vi "Build IPK Post Build.vi"(5 "Files Generated by Build":path[](array[path]), 6 "Top Level/Always Included VIs":path[](array[path]), 7 "Destination Path":path, 8 "error in (no error)":errorcluster, 9 "Target Name":string, 10 "Build Specification Name":string, 11 "Project Path":path) -> (0 "error out":errorcluster)   [LabVIEW 2013]
uses:
  <vilib>/AppBuilder/AB_API/common/AB_API Build Object Type.ctl
  <vilib>/AppBuilder/AB_Classes/RTEXE/AB_RTEXE.lvclass
  <vilib>/AppBuilder/AB_Classes/Build/AB_Build.lvclass
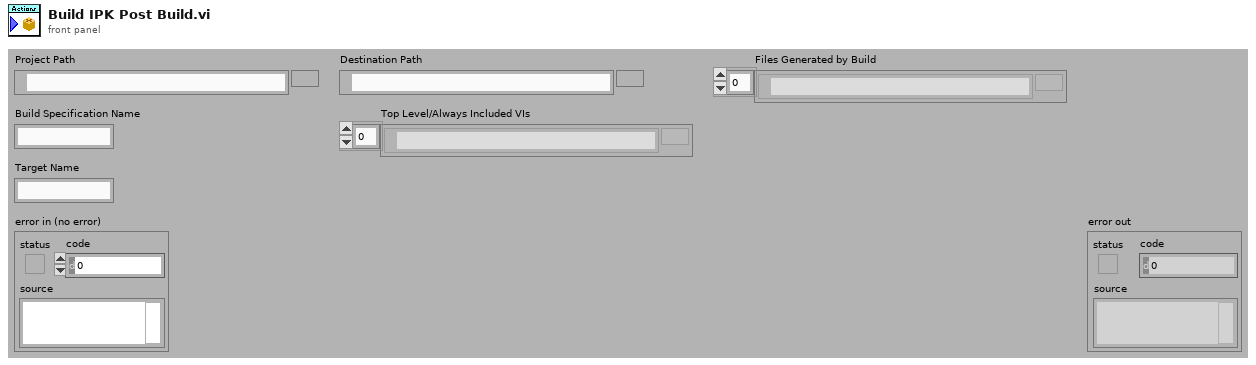
[diagram p1: front panel]
types:
  T1 = typedef "AB_API Build Object Type.ctl" = enum16{"Source Distribution", "DLL", "EXE", "Installer", "Zip File", "RESTful WS", "RTEXE", "Packed Library", "C Generation "}
  T2 = typedef "ItemRef.ctl" = u64
  T3 = typedef "AB_Build.ctl" = cluster{"buildSpecName":string, "buildSpecDescription":string, "destinations":refnum<class "AB_Destination.lvclass">[], "exclusionOption":T4, "defaultLanguage":string, "supportedLanguages":string[], "excludedDirectories":path[], "buildContext":refnum<vi>, "buildObject":T2, "preview":bool, "programatic":bool, "progressBarEvents":T5, "userLog_Path":path, "preActionID":string, "preAction_Path":path, "postActionID":string, "postAction_Path":path, "eng_checkForBrokenVIs?":bool, "eng_verboseLinkerErrors?":bool, "localDest_Path":path, "targetDest_Path":path, "removeVIObject":bool, "cache":refnum<class "PreviewCache.lvclass">, "use cache":bool, "previewCache_ID":string, "buildCache_ID":string, "eng_TempLocalDest_Path":path, "compilerOptimizationLevel":u32, "eng_collectDependencies?":bool, "versionInfo":cluster{"buildVersion":cluster{"major":u16, "minor":u16, "patch":u16, "build":u16}, "autoIncrement":bool}, "eng_enableVIChecksums":bool}
  T4 = typedef "AB_Exclusion_Option.ctl" = cluster{"typedefs":bool, "polymorphicVIs":bool, "unusedLibraryItems":bool, "modifyLibraryFile":bool, "edit-timeDependencies":bool, "inlineVIs":bool}
  T5 = typedef "provcom_ProgressBar_Events.ctl" = cluster{"newJob":refnum<user-event>, "newItem":refnum<user-event>, "errorMsg":T6, "cancel":refnum<user-event>}
  T6 = typedef "mxLvBuildError.ctl" = refnum<user-event>
  T7 = enum32{"invalid CPU target", "Motorola 68K", "PowerPC", "Intel x86", "SPARC", "PA-RISC", "MIPS", "Alpha", "ARM", "AMD/Intel x64"}
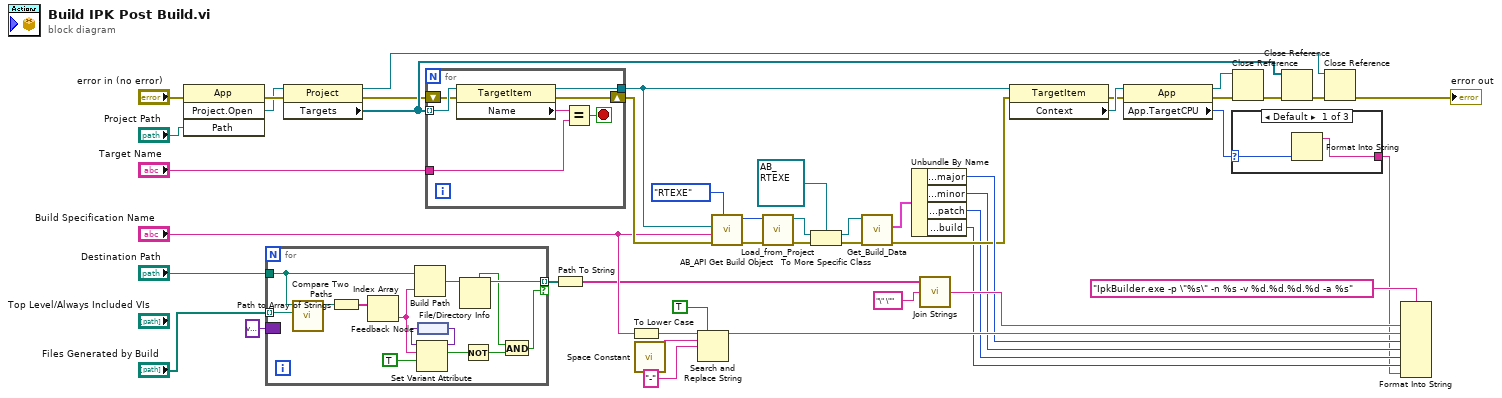
[diagram p0: block diagram]
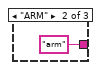
[diagram p2: hidden frame]
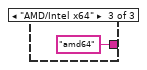
[diagram p3: hidden frame]
diagram:
  n1 = invoke class="App" method="Project.Open"(error in="error in (no error)", "Path"="Project Path") -> (error out=w44:errorcluster, "Project:Open"=w27:refnum<vi>)  [unwired: 2 in, 2 out]
  n2 = for {
    tunnel: "Files Generated by Build" -> [w61] mode=indexing
    tunnel: "Destination Path" -> [w58]
    tunnel: [w50] -> w13 mode=indexing if=w49
    border: variant -> [_]
    n3 = call <vilib>:"Compare Two Paths.vi"("Path 2"=w61, "Path 1"=w58) -> ("Relative Path from 1 to 2"=w60:path)  [unwired: 6 in, 3 out]
    n4 = Path to Array of Strings(0:w60) -> (2:w59:string[])  [unwired: 1 out]
    n5 = Index Array(array=w59) -> (element=w57:string)  [unwired: 1 in]
    n6 = Build Path(base path=w58, name or relative path=w57) -> (appended path=w51:path)
    n7 = feedback #1() -> (w52:variant)
    n8 = Set Variant Attribute(Variant=w52, name=w57, value=TRUE) -> (Variant out=w53:variant, replaced=w55:bool)  [unwired: 1 in, 1 out]
    n9 = feedback-in #1(w53) -> ()
    n10 = File/Directory Info(path=w51) -> (path out=w50:path, directory=w48:bool)  [unwired: 1 in, 5 out]
    n11 = Not(x=w55) -> (.not. x?=w54:bool)
    n12 = And(x=w48, y=w54) -> (x .and. y?=w49:bool)
  }
  n13 = property class="Project"(reference=w27, error in=w44) -> (reference out=w35:refnum<vi>, error out=w38:errorcluster, "Targets"=w42:refnum<vi>[])
  n14 = for {
    tunnel: w42 -> [w68] mode=indexing
    shift-right: [w64] -> w37
    shift-left: w38 -> [w67]
    tunnel: "Target Name" -> [w65]
    tunnel: [w63] -> w26
    stop <- w62 stop-if-true
    n15 = property class="TargetItem"(reference=w68, error in=w67) -> (reference out=w63:refnum<vi>, error out=w64:errorcluster, "Name"=w66:string)
    n16 = Equal?(x=w66, y=w65) -> (x = y?=w62:bool)
  }
  n17 = Path To String(path=w13) -> (string=w12:string[])
  n18 = To Lower Case(string="Build Specification Name") -> (all lower case string=w18:string)
  n19 = call <vilib>:"Space Constant.vi"() -> ("String"=w17:string)
  n20 = Search and Replace String(replace all?=TRUE ("replace all? (F)"), input string=w18, search string=w17, replace string="-" ("replace string (\"\")")) -> (result string=w9:string)  [unwired: 4 in, 3 out]
  n21 = call <vilib>:"AB_API Get Build Object.vi"("Build object type"=AB_API_Build_Object_Type."RTEXE", "error in (no error)"=w37, "Build spec name"="Build Specification Name", "TargetItem Refnum"=w26) -> ("error out"=w39:errorcluster, "Build Object"=w40:T2)  [unwired: 1 in, 5 out]
  n22 = call <vilib>:"Load_from_Project.vi"("error in (no error)"=w39, "Object"=w40) -> ("error out"=w34:errorcluster, "Build out"=w33:refnum<class "AB_Build.lvclass">)  [unwired: 8 out]
  n23 = To More Specific Class(target class=refnum<class "AB_RTEXE.lvclass"> refnum ("AB_RTEXE.lvclass"), reference=w33, error in=w34) -> (specific class reference=w31:refnum<class "AB_RTEXE.lvclass">, error out=w30:errorcluster)
  n24 = call <vilib>:"Get_Build_Data.vi"("error in (no error)"=w30, "Class in"=w31) -> ("error out"=w7:errorcluster, "data"=w29:T3)  [unwired: 7 in, 1 out]
  n25 = Unbundle By Name(w29) -> ("versionInfo.buildVersion.major"=w8:u16, "versionInfo.buildVersion.minor"=w4:u16, "versionInfo.buildVersion.patch"=w5:u16, "versionInfo.buildVersion.build"=w6:u16)
  n26 = call <vilib>:"Join Strings.vi"("Separator (,)"="\" \"", "Strings In"=w12) -> ("String"=w10:string)  [unwired: 1 in]
  n27 = property class="TargetItem"(reference=w26, error in=w7) -> (error out=w22:errorcluster, "Context"=w25:refnum<vi>)  [unwired: 1 out]
  n28 = property class="App"(reference=w25, error in=w22) -> (reference out=w23:refnum<vi>, error out=w24:errorcluster, "App.TargetCPU"=w20:T7)
  n29 = case shown="Default" w20 {
    selector: w20 -> [w70 _ _]
    tunnel: [w69 "arm" "amd64"] -> w3
    frame Default {
      n30 = Format Into String(w70) -> (resulting string=w69:string)  [unwired: 3 in, 1 out]
    }
    frame "ARM" {
    }
    frame "AMD/Intel x64" {
    }
  }
  n31 = Close Reference(reference=w23, error in (no error)=w24) -> (error out=w21:errorcluster)
  n32 = Close Reference(reference=w42, error in (no error)=w21) -> (error out=w36:errorcluster)
  n33 = Close Reference(reference=w35, error in (no error)=w36) -> (error out=→"error out":errorcluster)
  n34 = Format Into String(format string="IpkBuilder.exe -p \"%s\" -n %s -v %d.%d.%d.%d -a %s", w10, w9, w8, w4, w5, w6, w3) -> ()  [unwired: 2 in, 2 out]
